vi "攻击盘.vi"() -> ()   [LabVIEW 2013]
panel:
  in  "普通8":bool
  in  "普通7":bool
  in  "普通6":bool
  in  "普通5":bool
  in  "普通4":bool
  in  "普通3":bool
  in  "普通2":bool
  in  "普通1":bool
  in  "状态":T1(ring)
  in  "攻击簇":cluster{"普通攻击":bool, "投掷攻击":bool, "返回":bool}
  in  "停止":bool
  in  "逃跑":bool
  in  "物品":bool
  in  "仙术":bool
  in  "攻击":bool
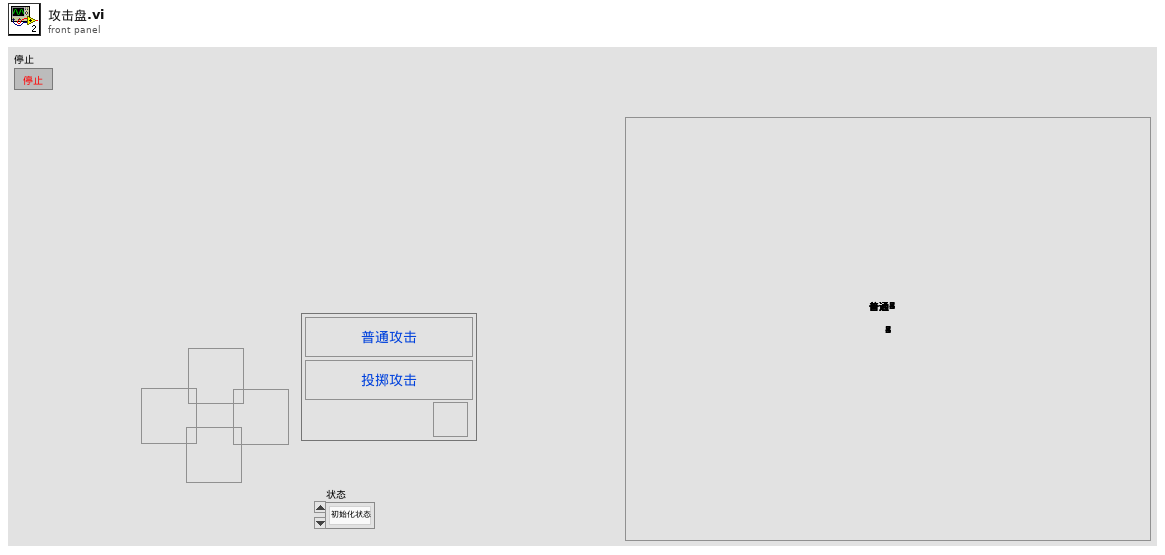
[diagram p1: front panel]
types:
  T1 = enum16{"初始化状态", "结束状态", "撤销状态", "偷窃", "逃跑", "--设置--", "还神丹", "止血草", "--物品--", "投掷攻击", "普通攻击", "--攻击--", "雷咒", "风咒", "炎咒", "--仙术--", "行动盘状态", "我方攻击状态", "敌人攻击状态", "时间条状态"}
  T2 = cluster{bool, bool, bool, bool, bool, bool, bool, bool}
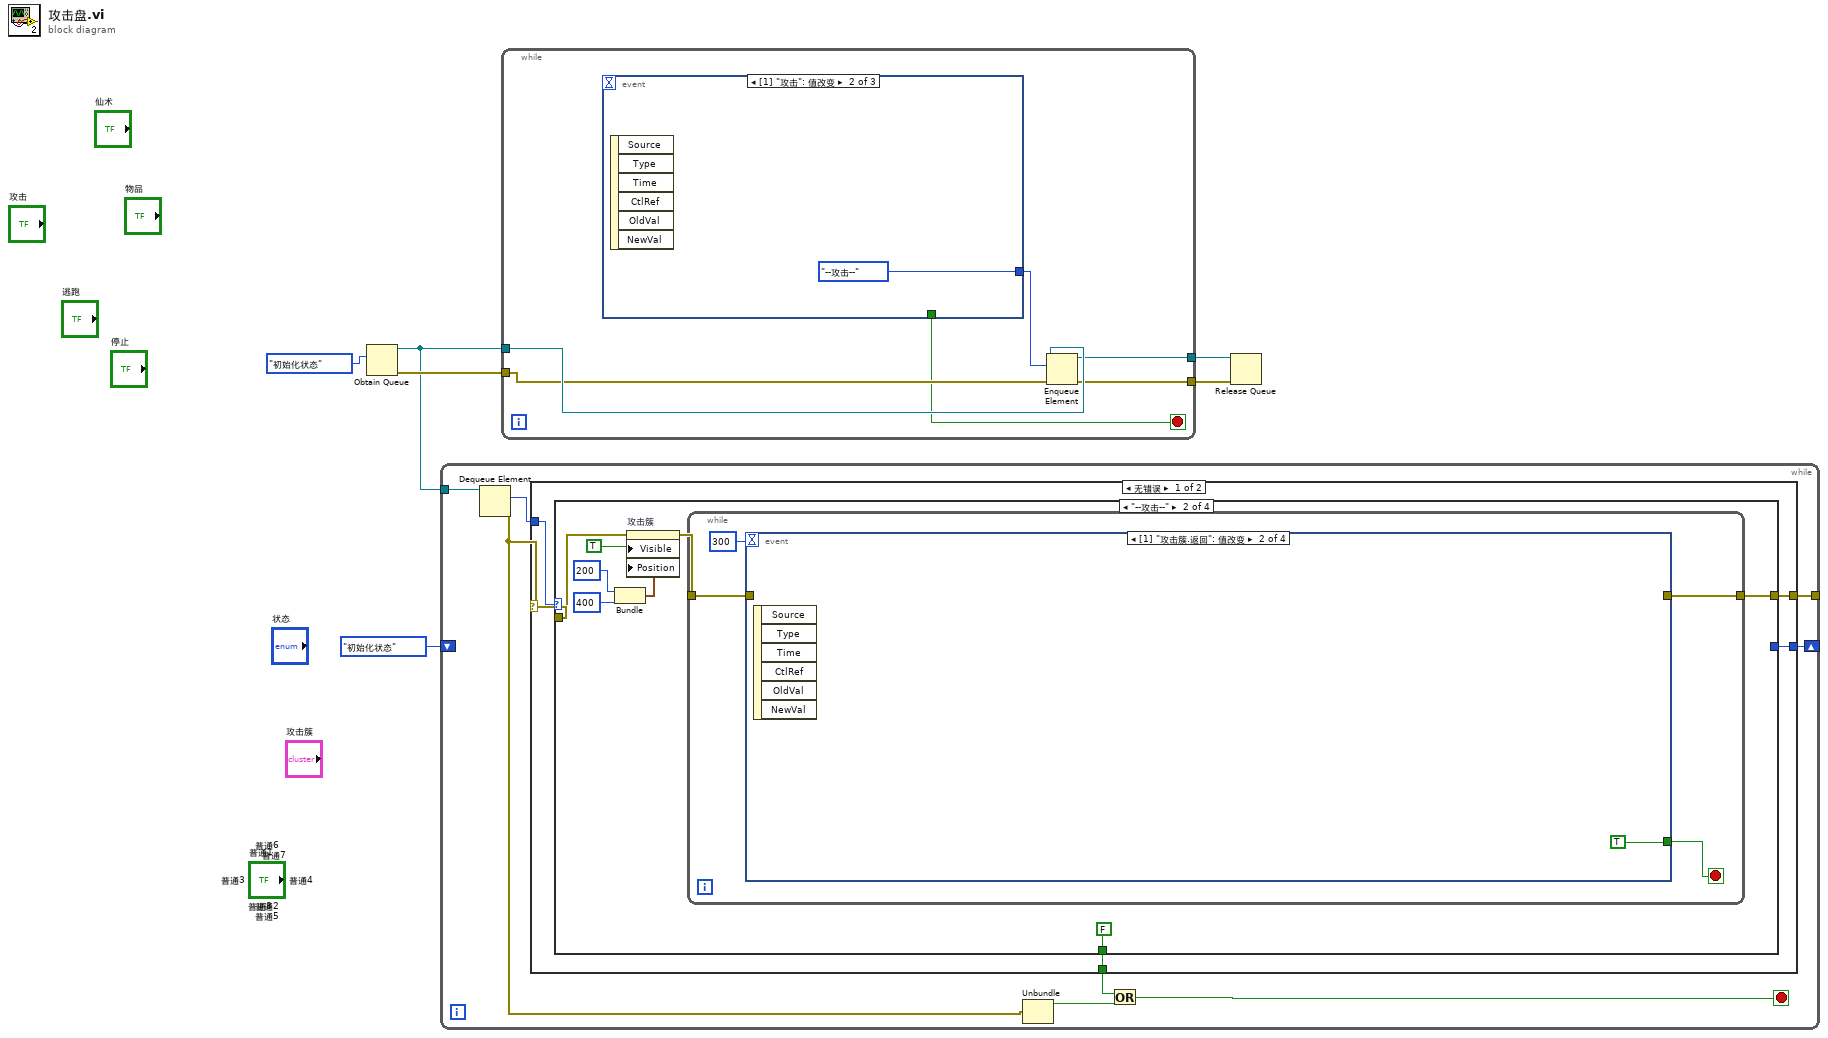
[diagram p0: block diagram]
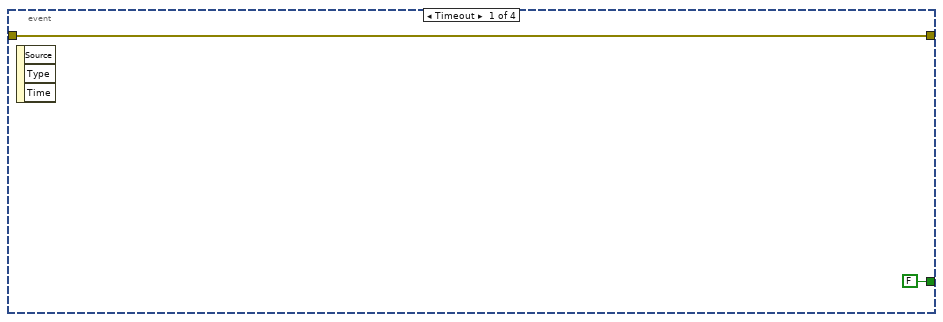
[diagram p3: hidden frame]
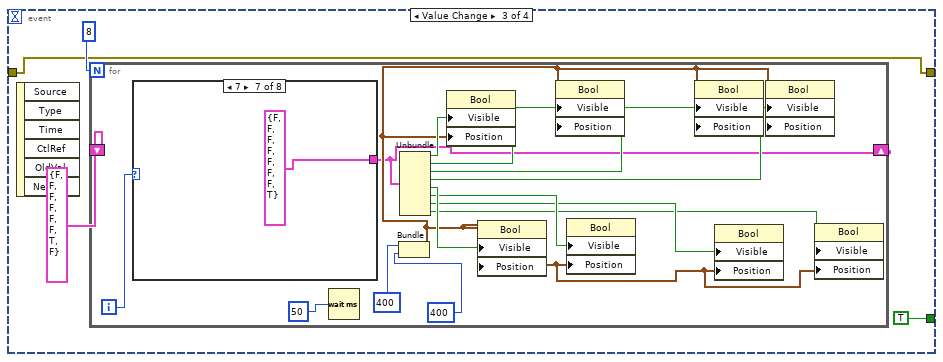
[diagram p4: hidden frame]
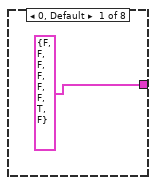
[diagram p5: hidden frame]
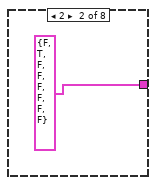
[diagram p6: hidden frame]
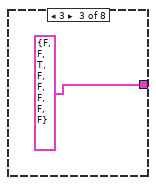
[diagram p7: hidden frame]
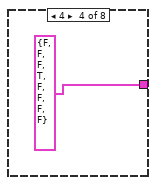
[diagram p8: hidden frame]
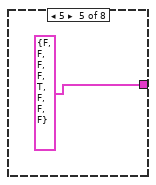
[diagram p9: hidden frame]
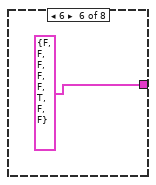
[diagram p10: hidden frame]
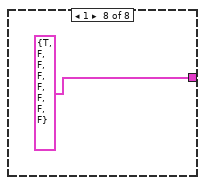
[diagram p11: hidden frame]
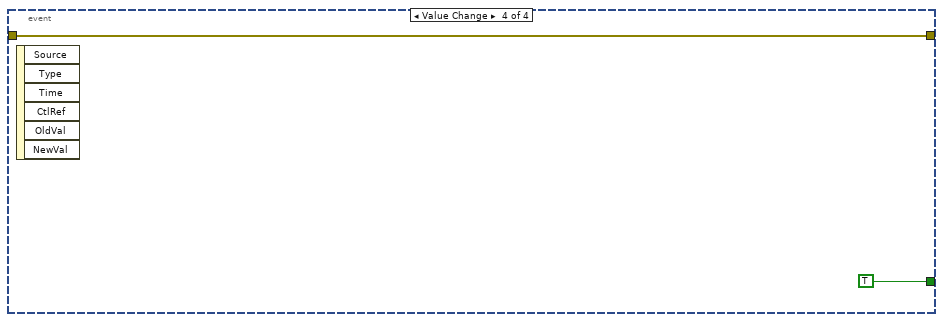
[diagram p12: hidden frame]
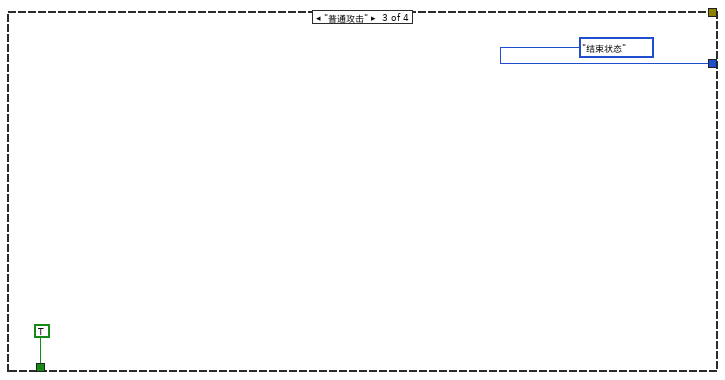
[diagram p13: hidden frame]
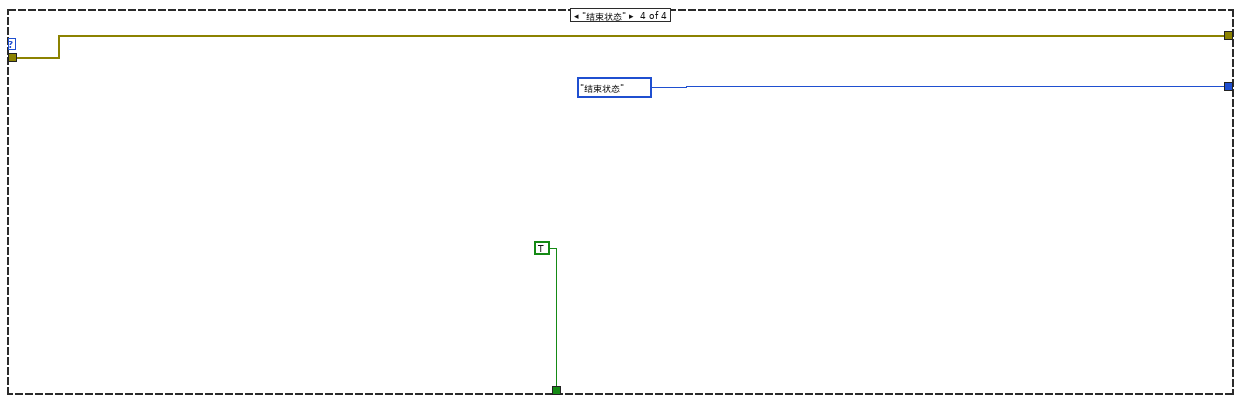
[diagram p14: hidden frame]
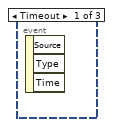
[diagram p16: hidden frame]
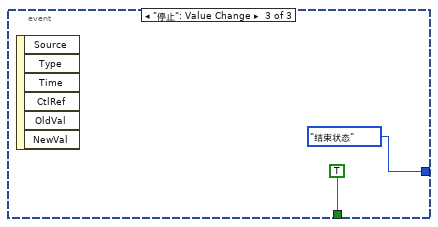
[diagram p17: hidden frame]
diagram:
  n1 = Obtain Queue(element data type=T1."初始化状态" ("状态")) -> (queue out=w2:refnum<queue>, error out=w6:errorcluster)  [unwired: 4 in, 1 out]
  n2 = while {
    tunnel: w2 -> [w14]
    shift-right: [w12] -> _
    shift-left: T1."初始化状态" ("状态") -> [_]
    tunnel: [w11] -> _
    stop <- w7 stop-if-true
    n3 = Dequeue Element(queue=w14) -> (element=w13:T1, error out=w10:errorcluster)  [unwired: 2 in, 2 out]
    n4 = case shown="无错误" w10 {
      selector: w10 -> [w19 _]
      tunnel: w13 -> [w15 _]
      tunnel: [w18 _] -> w12
      tunnel: [w17 _] -> w11
      tunnel: [w16 _] -> w8
      frame No Error {
        n5 = case shown="\"--攻击--\"" w15 {
          tunnel: w19 -> [_ w23 _ w67]
          tunnel: [_ _ T1."结束状态" ("状态") T1."结束状态" ("状态")] -> w18
          tunnel: [_ w21 _ w67] -> w17
          tunnel: [_ FALSE TRUE TRUE] -> w16
          frame "初始化状态", Default {
          }
          frame "--攻击--" {
            n6 = Bundle(200, 400) -> (w24:cluster{i32, i32})  [unwired: 1 in]
            n7 = property on="攻击簇" class="Clust"(error in=w23, "Visible"=TRUE, "Position"=w24) -> (error out=w22:errorcluster)  [unwired: 1 in, 1 out]
            n8 = while {
              tunnel: w22 -> [w31]
              tunnel: [w29] -> w21
              stop <- w28 stop-if-true
              n9 = event shown="[1] \"攻击簇.返回\": 值改变" {
                selector: _ -> [_ _ _ _]
                dyn-events: _ -> [_ _ _ _]
                timeout: 300 -> [_ _ _ _]
                tunnel: w31 -> [w33 _ w35 w61]
                tunnel: [w33 _ w35 w61] -> w29
                tunnel: [FALSE TRUE TRUE TRUE] -> w28
                event Timeout {
                  n10 = event-data() -> ()  [unwired: 1 in, 3 out]
                }
                event "攻击簇.返回": Value Change {
                  n11 = event-data() -> ()  [unwired: 1 in, 6 out]
                }
                event "攻击簇.普通攻击": Value Change {
                  n12 = event-data() -> ()  [unwired: 1 in, 6 out]
                  n13 = for {
                    N: 8 -> [_]
                    shift-right: [w40] -> _
                    shift-left: T2 {FALSE, FALSE, FALSE, FALSE, FALSE, FALSE, TRUE, FALSE} -> [_]
                    i -> [w52]
                    n14 = case shown="7" w52 {
                      tunnel: [T2 {FALSE, FALSE, FALSE, FALSE, FALSE, FALSE, TRUE, FALSE} T2 {FALSE, TRUE, FALSE, FALSE, FALSE, FALSE, FALSE, FALSE} T2 {FALSE, FALSE, TRUE, FALSE, FALSE, FALSE, FALSE, FALSE} T2 {FALSE, FALSE, FALSE, TRUE, FALSE, FALSE, FALSE, FALSE} T2 {FALSE, FALSE, FALSE, FALSE, TRUE, FALSE, FALSE, FALSE} T2 {FALSE, FALSE, FALSE, FALSE, FALSE, TRUE, FALSE, FALSE} T2 {FALSE, FALSE, FALSE, FALSE, FALSE, FALSE, FALSE, TRUE} T2 {TRUE, FALSE, FALSE, FALSE, FALSE, FALSE, FALSE, FALSE}] -> w40
                      frame 0, Default {
                      }
                      frame 2 {
                      }
                      frame 3 {
                      }
                      frame 4 {
                      }
                      frame 5 {
                      }
                      frame 6 {
                      }
                      frame 7 {
                      }
                      frame 1 {
                      }
                    }
                    n15 = Wait (ms)(milliseconds to wait=u32 50 ("毫秒倍数")) -> ()  [unwired: 1 out]
                    n16 = Bundle(400, 400) -> (w41:cluster{i32, i32})  [unwired: 1 in]
                    n17 = Unbundle(w40) -> (w51:bool, w50:bool, w49:bool, w48:bool, w47:bool, w46:bool, w45:bool, w44:bool)
                    n18 = property on="属性节点" class="Bool"("Visible"=w51, "Position"=w41) -> ()  [unwired: 2 in, 2 out]
                    n19 = property on="属性节点" class="Bool"("Visible"=w47, "Position"=w41) -> ()  [unwired: 2 in, 2 out]
                    n20 = property on="属性节点" class="Bool"("Visible"=w50, "Position"=w41) -> ()  [unwired: 2 in, 2 out]
                    n21 = property on="属性节点" class="Bool"("Visible"=w46, "Position"=w41) -> ()  [unwired: 2 in, 2 out]
                    n22 = property on="属性节点" class="Bool"("Visible"=w49, "Position"=w41) -> ()  [unwired: 2 in, 2 out]
                    n23 = property on="属性节点" class="Bool"("Visible"=w45, "Position"=w41) -> ()  [unwired: 2 in, 2 out]
                    n24 = property on="属性节点" class="Bool"("Visible"=w48, "Position"=w41) -> ()  [unwired: 2 in, 2 out]
                    n25 = property on="属性节点" class="Bool"("Visible"=w44, "Position"=w41) -> ()  [unwired: 2 in, 2 out]
                  }
                }
                event "攻击簇.投掷攻击": Value Change {
                  n26 = event-data() -> ()  [unwired: 1 in, 6 out]
                }
              }
            }
          }
          frame "普通攻击" {
          }
          frame "结束状态" {
          }
        }
      }
      frame Error {
      }
    }
    n27 = Unbundle(w10) -> ("status"=w9:bool)  [unwired: 2 out]
    n28 = Or(x=w8, y=w9) -> (x .or. y?=w7:bool)
  }
  n29 = while {
    tunnel: w2 -> [w73]
    tunnel: w6 -> [w70]
    tunnel: [w71] -> w4
    tunnel: [w69] -> w3
    stop <- w68 stop-if-true
    n30 = event shown="[1] \"攻击\": 值改变" {
      selector: _ -> [_ _ _]
      dyn-events: _ -> [_ _ _]
      timeout: _ -> [_ _ _]
      tunnel: [_ T1."--攻击--" ("状态") T1."结束状态" ("状态")] -> w72
      tunnel: [_ _ TRUE] -> w68
      event Timeout {
        n31 = event-data() -> ()  [unwired: 1 in, 3 out]
      }
      event "攻击": Value Change {
        n32 = event-data() -> ()  [unwired: 1 in, 6 out]
      }
      event "停止": Value Change {
        n33 = event-data() -> ()  [unwired: 1 in, 6 out]
      }
    }
    n34 = Enqueue Element(queue=w73, element=w72, error in (no error)=w70) -> (queue out=w71:refnum<queue>, error out=w69:errorcluster)  [unwired: 1 in, 1 out]
  }
  n35 = Release Queue(queue=w4, error in (no error)=w3) -> ()  [unwired: 1 in, 3 out]
